vi "Queue Example.vi"() -> ()   [LabVIEW 2020]
uses:
  Source/Type Defs/Debug Level.ctl
  Source/Sinks/Queue Sink/Queue Sink.lvclass
  C:/Users/hughe_cx/Documents/05_repos/LVLog/Source/Sinks/Sink/Sink.lvclass
  Source/LV Log.lvlib
  Source/Logger/Logger.lvclass
panel:
  out "created new?":bool
  out "Log Output":string[](array[string])
  in  "error in (no error)":errorcluster
  in  "Debug Level":T1=enum."DEBUG"
  out "error out":errorcluster
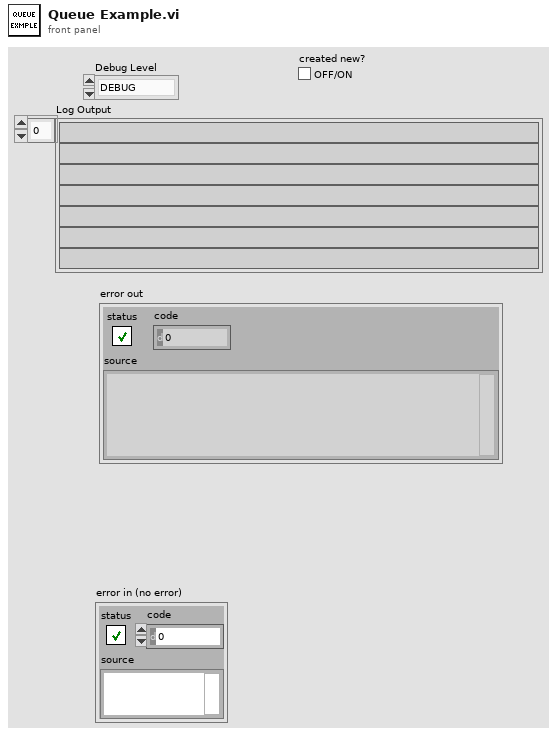
[diagram p1: front panel]
types:
  T1 = typedef "LV Log.lvlib/Debug Level.ctl" = enum16{"DEFAULT", "DEBUG", "INFO", "WARN", "ERROR", "FATAL"}
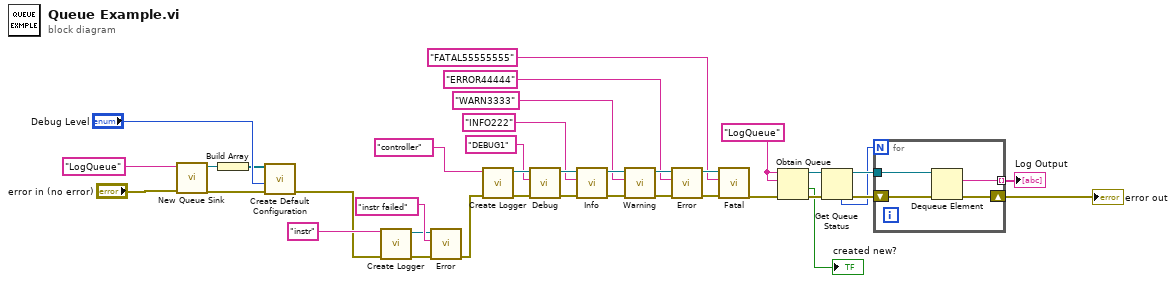
[diagram p0: block diagram]
diagram:
  w5 = "LogQueue" ("name (unnamed)")
  n1 = call "New Queue Sink.vi"("error in (no error)"="error in (no error)", "Queue Name"="LogQueue") -> ("error out"=w17:errorcluster, "Queue Sink out"=w2:refnum<class "Queue Sink.lvclass">)  [unwired: 8 in]
  n2 = Build Array(w2) -> (w1:refnum<class "Queue Sink.lvclass">[])
  n3 = call "Create Default Configuration.vi"("Sinks"=w1, "Debug Level in"="Debug Level", "error in (no error)"=w17) -> ("error out"=w15:errorcluster)  [unwired: 7 in]
  n4 = call "Create Logger.vi"("error in (no error)"=w15, "Name"="instr") -> ("error out"=w19:errorcluster, "Logger out"=w20:refnum<class "Logger.lvclass">)  [unwired: 8 in]
  n5 = call "Error.vi"("error in (no error)"=w19, "Log Text"="instr failed", "Logger in"=w20) -> ("error out"=w21:errorcluster)  [unwired: 6 in, 2 out]
  n6 = call "Create Logger.vi"("error in (no error)"=w21, "Name"="controller") -> ("error out"=w37:errorcluster, "Logger out"=w36:refnum<class "Logger.lvclass">)  [unwired: 8 in]
  n7 = call "Debug.vi"("error in (no error)"=w37, "Log Text"="DEBUG1", "Logger in"=w36) -> ("error out"=w34:errorcluster, "Logger out"=w35:refnum<class "Logger.lvclass">)  [unwired: 6 in, 1 out]
  n8 = call "Info.vi"("error in (no error)"=w34, "Log Text"="INFO222", "Logger in"=w35) -> ("error out"=w33:errorcluster, "Logger out"=w32:refnum<class "Logger.lvclass">)  [unwired: 6 in, 1 out]
  n9 = call "Warning.vi"("error in (no error)"=w33, "Log Text"="WARN3333", "Logger in"=w32) -> ("error out"=w30:errorcluster, "Logger out"=w31:refnum<class "Logger.lvclass">)  [unwired: 6 in, 1 out]
  n10 = call "Error.vi"("error in (no error)"=w30, "Log Text"="ERROR44444", "Logger in"=w31) -> ("error out"=w29:errorcluster, "Logger out"=w28:refnum<class "Logger.lvclass">)  [unwired: 6 in, 1 out]
  n11 = call "Fatal.vi"("error in (no error)"=w29, "Log Text"="FATAL55555555", "Logger in"=w28) -> ("error out"=w9:errorcluster)  [unwired: 6 in, 2 out]
  n12 = Obtain Queue(name (unnamed)=w5, element data type=w5, error in (no error)=w9) -> (queue out=w11:refnum<queue>, created new?=→"created new?":bool, error out=w10:errorcluster)  [unwired: 2 in]
  n13 = Get Queue Status(queue=w11, error in (no error)=w10) -> (queue out=w7:refnum<queue>, error out=w8:errorcluster, # elements in queue=w3:i32)  [unwired: 1 in, 5 out]
  n14 = for {
    N: w3 -> [_]
    shift-right: [w40] -> w12
    shift-left: w8 -> [w42]
    tunnel: w7 -> [w41]
    tunnel: [w39] -> w6 mode=indexing
    n15 = Dequeue Element(queue=w41, error in (no error)=w42) -> (element=w39:string, error out=w40:errorcluster)  [unwired: 1 in, 2 out]
  }
  "error out" <- w12
  "Log Output" <- w6
